vi "UpdateRoiLimits.vi"(0 "object in":refnum<class "Hamamatsu.lvclass">, 1 "reference to front panel item":refnum<vi>, 2 "SubRegionLimits":T2 {"V Size"."Value" min=0 max=0 step=4; "H Size"."Value" min=0 max=0 step=4; "V Offset"."Value" min=0 max=0 step=4; "H Offset"."Value" min=0 max=0 step=4}, 5 "error in (no error)":errorcluster) -> (14 "object out":refnum<class "Hamamatsu.lvclass">, 19 "error out":errorcluster)   [LabVIEW 2019, in "Hamamatsu.lvclass"]
uses:
  Hamamatsu.lvclass
  <vilib>/Utility/miscctls.llb/LVMinMaxIncTypeDef.ctl
panel:
  in  "Sub Region Placeholder":T3
  out "error out 2":errorcluster
  in  "error in (no error) 2":errorcluster
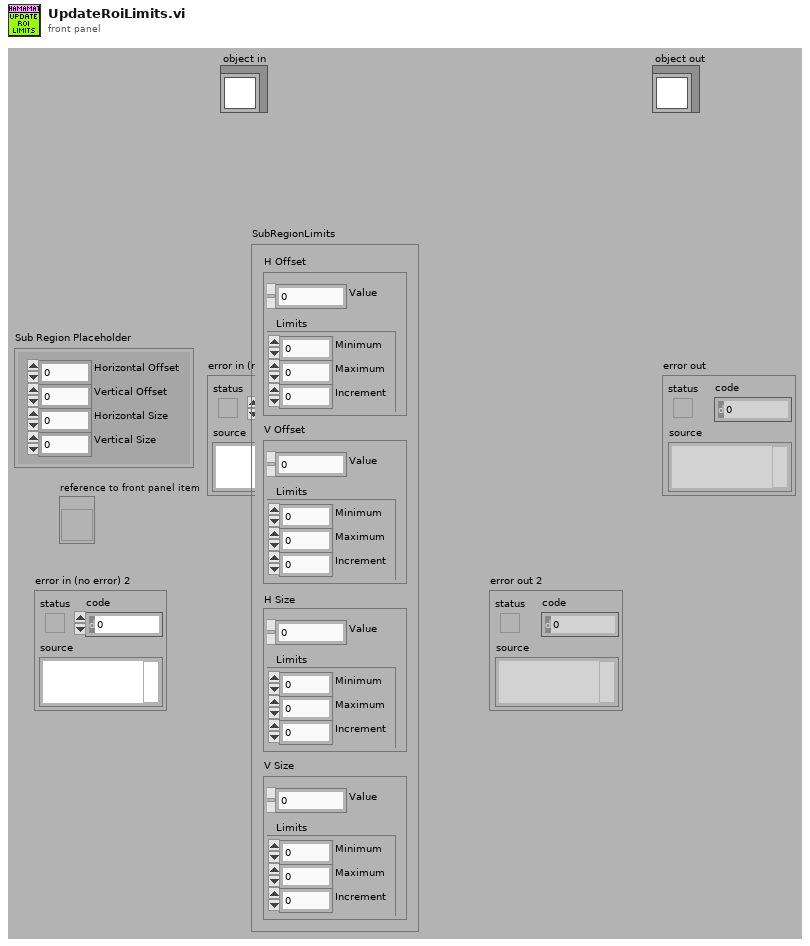
[diagram p1: front panel]
types:
  T1 = typedef "LVMinMaxIncTypeDef.ctl" = cluster{"Minimum":dbl, "Maximum":dbl, "Increment":dbl}
  T2 = cluster{"H Offset":cluster{"Value":i32, "Limits":T1}, "V Offset":cluster{"Value":i32, "Limits":T1}, "H Size":cluster{"Value":i32, "Limits":T1}, "V Size":cluster{"Value":i32, "Limits":T1}}
  T3 = cluster{"Horizontal Offset":i32, "Vertical Offset":i32, "Horizontal Size":i32, "Vertical Size":i32}
  T4 = cluster{"Out of Range Action Minimum":u8, "Out of Range Action Maximum":u8, "Out of Range Action Increment":u8}
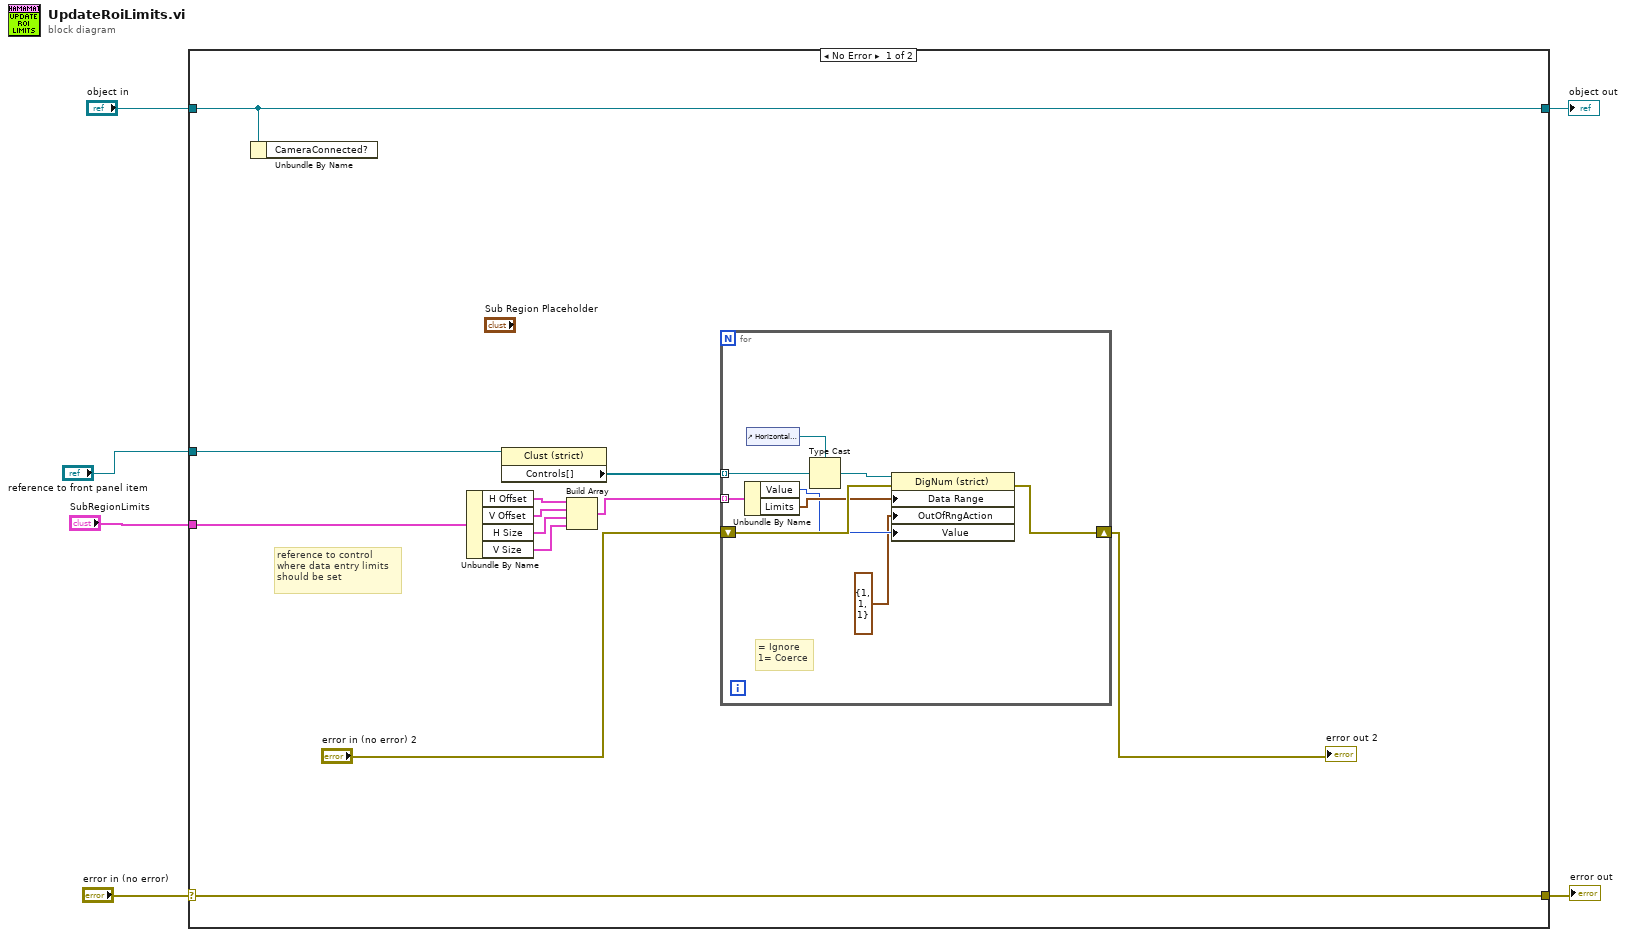
[diagram p0: block diagram]
diagram:
  n1 = case shown="No Error" "error in (no error)" {
    selector: "error in (no error)" -> [w18 w29]
    tunnel: [w18 w29] -> w5
    tunnel: [w17 w28] -> w3
    tunnel: "object in" -> [w17 w28]
    tunnel: "SubRegionLimits" -> [w8 _]
    tunnel: "reference to front panel item" -> [w7 _]
    frame No Error {
      # "reference to control\nwhere data entry limits \nshould be set"
      n2 = Unbundle By Name(w17) -> ()  [unwired: 1 out]
      n3 = Unbundle By Name(w8) -> ("H Offset"=w13:cluster{"Value":i32, "Limits":T1}, "V Offset"=w11:cluster{"Value":i32, "Limits":T1}, "H Size"=w10:cluster{"Value":i32, "Limits":T1}, "V Size"=w9:cluster{"Value":i32, "Limits":T1})
      n4 = property on="Property Node" class="Clust (strict)"(reference=w7) -> ("Controls[]"=w14:refnum<vi>[])  [unwired: 1 in, 2 out]
      n5 = Build Array(w13, w11, w10, w9) -> (w12:cluster{"Value":i32, "Limits":T1}[])
      n6 = for {
        tunnel: w14 -> [w26] mode=indexing
        tunnel: w12 -> [w22] mode=indexing
        shift-right: [w24] -> w15
        shift-left: "error in (no error) 2" -> [w25]
        # "= Ignore\n1= Coerce"
        n7 = Unbundle By Name(w22) -> ("Value"=w20:i32, "Limits"=w21:T1)
        n8 = control-ref of="Horizontal Offset"() -> (w27:refnum<vi>)
        n9 = Type Cast(type=w27, x=w26) -> (*(type *) &x=w23:refnum<vi>)
        n10 = property on="Property Node" class="DigNum (strict)"(reference=w23, error in=w25, "Data Range"=w21, "OutOfRngAction"=T4 {"Out of Range Action Minimum"=1, "Out of Range Action Maximum"=1, "Out of Range Action Increment"=1} ("Response to Value Outside Limits"), "Value"=w20) -> (error out=w24:errorcluster)  [unwired: 1 out]
      }
      "error out 2" <- w15
    }
    frame Error {
    }
  }
  "error out" <- w5
  "object out" <- w3
